vi "setSampling(private).vi"(8 "error in (no error)":errorcluster, 10 "Sampling":T1={"Fs"=204789.0, "#s"=15753} {"Fs" format="%#_13g"}, 11 "DAQmx in":refnum<class "DAQmx.lvclass">) -> (0 "error out":errorcluster, 3 "DAQmx out":refnum<class "DAQmx.lvclass">)   [LabVIEW 2019, in "DAQmx.lvclass"]
uses:
  DAQmx.lvclass
  DAQmx.lvclass/DAQmx.ctl
  typedefs/DAQ.Config.Timing.Sampling--Cluster.ctl
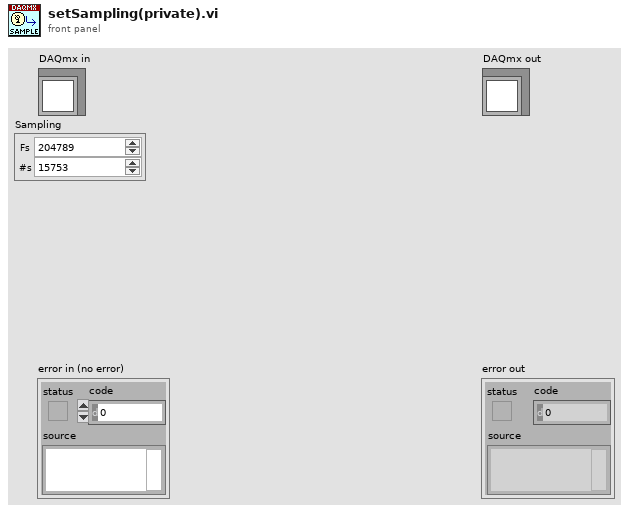
[diagram p1: front panel]
types:
  T1 = typedef "DAQmx.lvclass/DAQ.Config.Timing.Sampling--Cluster.ctl" = cluster{"Fs":dbl, "#s":i32}
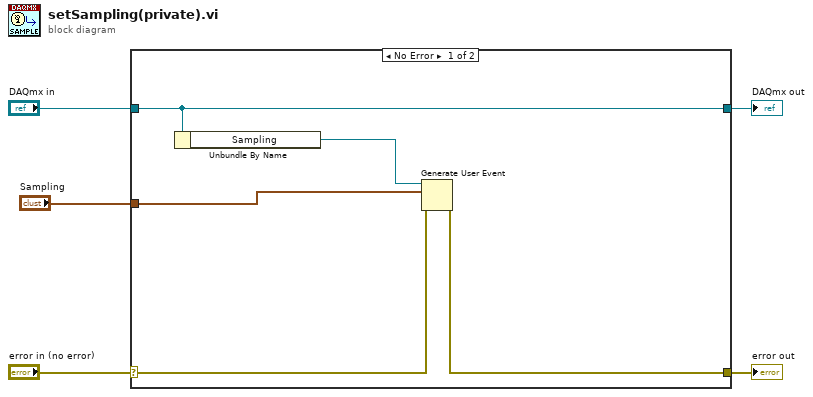
[diagram p0: block diagram]
diagram:
  n1 = case shown="No Error" "error in (no error)" {
    selector: "error in (no error)" -> [w8 w12]
    tunnel: [w7 w12] -> w4
    tunnel: [w10 w11] -> w2
    tunnel: "DAQmx in" -> [w10 w11]
    tunnel: "Sampling" -> [w6 _]
    frame No Error {
      n2 = Unbundle By Name(w10) -> ("Sampling"=w9:refnum<user-event>)
      n3 = Generate User Event(user event=w9, event data cluster=w6, error in=w8) -> (error out=w7:errorcluster)  [unwired: 1 in, 1 out]
    }
    frame Error {
    }
  }
  "error out" <- w4
  "DAQmx out" <- w2
